vi "SL9200 Driver SM.vi"(0 "ComPort":refnum<visa-resource-name>="COM1", 2 "Mode":enum16{"Read", "Write"}(ring), 5 "Register":T1=49 items=["Heat_Flow", "Mass_Flow", "Corrected_Volume_Flow", "Volume_Flow", "Temperature", "Temperature2", "Delta_Temperature", "Pressure", "Diff_Pressure", "Density", "Spec_Enthalpy", "Date", "Time", "Level", "Peak_Demand", "Demand_Last_Hour", "Peak_Demand_Time", "Peak_Demand_Date", "Viscosity", "Reynolds_Number", "Heat_Total", "Grand_Heat_Total", "Mass_Total", "Grand_Mass", "Corrected_Volume_Total", "Grand_Corrected_Volume", "Volume_Total", "Grand_Volume", "Totalizer_Reset", "Alarm_Reset", "Barometric", "Fluid_Type", "Reference_Density", "Therm_Expansion_Coef", "Combustion_Heat", "Specific_Heat", "Flow_Z_Factor", "Ref_Z_Factor", "Isentropic_Exponent", "Viscosity_A", "Viscosity_B", "Reference_Temperature", "Calibration_Density", "Base_Density_H2O_4C", "Per_Mole_N2", "Per_Mole_CO2", "Tag_Number", "Software_Version", "Hardware_Version", "Order_Code", "Serial_Number", "Sensor_Serial_Num"], 7 "Write Data":string, 9 "InitSerial?":bool=TRUE, 11 "Error In":errorcluster, 12 "Close Com":bool) -> (4 "CMD OK":bool, 6 "Response":string, 15 "Error Out":errorcluster)   [LabVIEW 2016]
uses:
  Type Definitions/SL9200 Registers.ctl
  <vilib>/Instr/_visa.llb/VISA Configure Serial Port (Instr).vi
panel:
  out "Command String":string
  out "tStart":u32
  out "Time Array":i32[](array[numeric])
  out "State Array":string[](array[string])
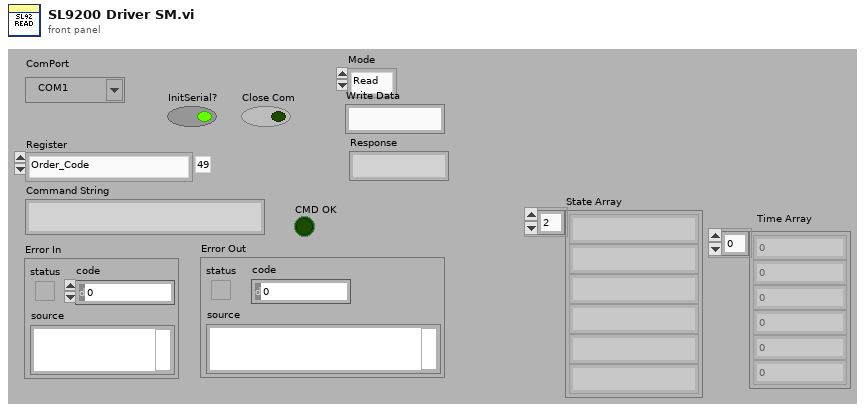
[diagram p1: front panel]
types:
  T1 = typedef "SL9200 Registers.ctl" = u8
  T2 = enum32{"invalid app kind", "Development System", "Run Time System", "Student Edition", "Embedded LabVIEW", "Evaluation", "Custom"}
  T3 = cluster{"Current VI Reference":refnum<vi>, "Close Panel on Exit?":bool}
  T4 = enum32{"Invalid", "Standard", "Closed", "Hidden", "Minimized", "Maximized"}
  T5 = cluster{"Core":cluster{"Current VI Reference":refnum<vi>, "Close Panel on Exit?":bool}, "ComPort":refnum<visa-resource-name>, "Response":string, "CMD OK":bool, "CMD":string, "Error Out Flag":bool}
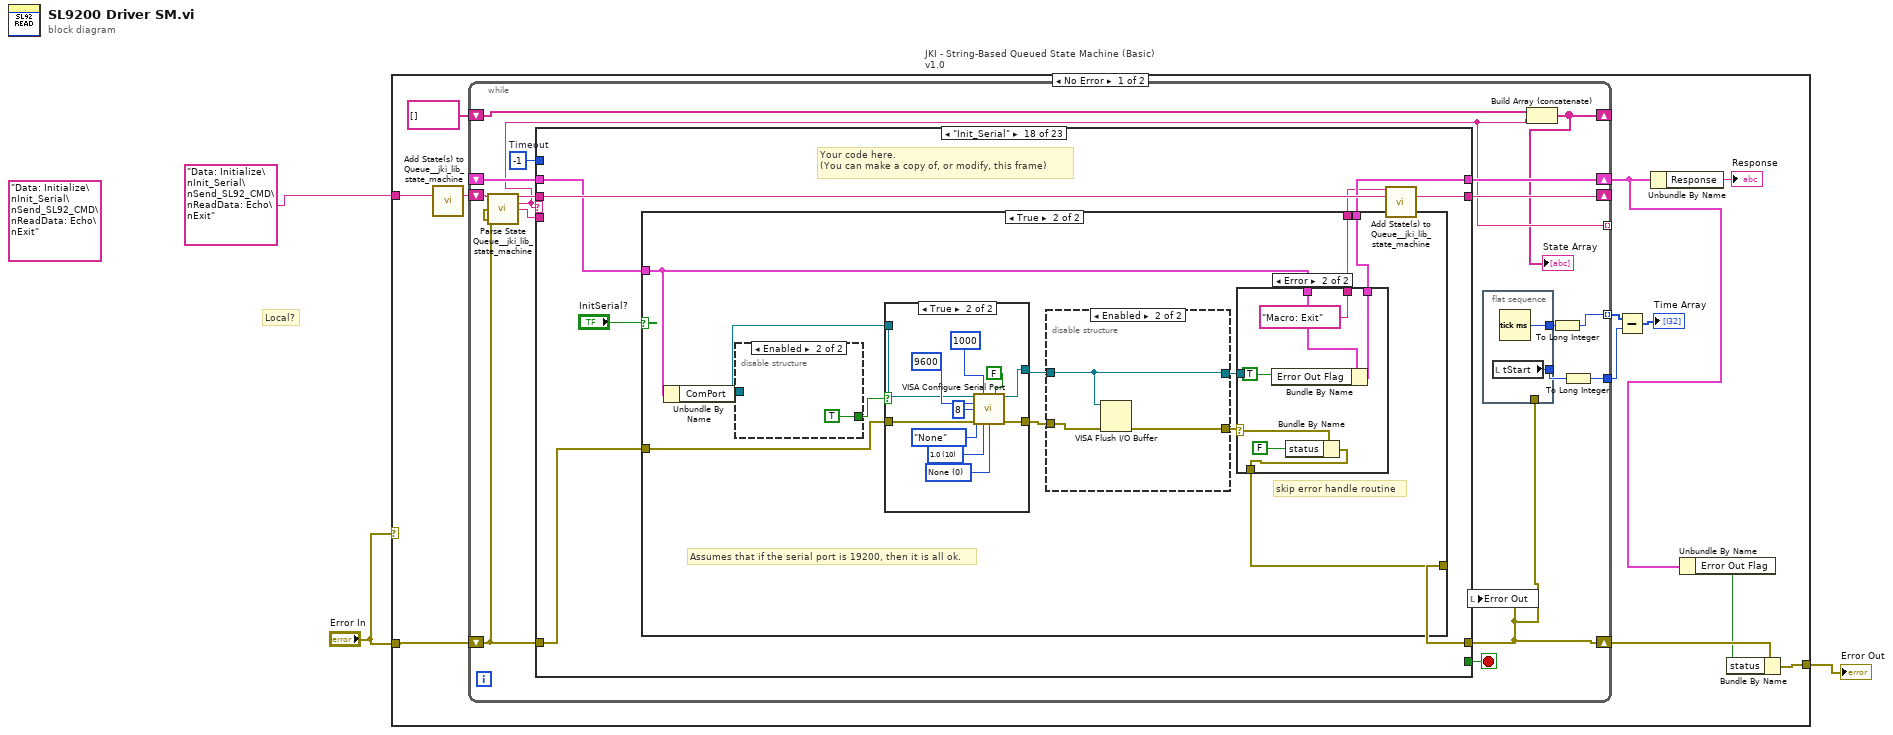
[diagram p0: block diagram]
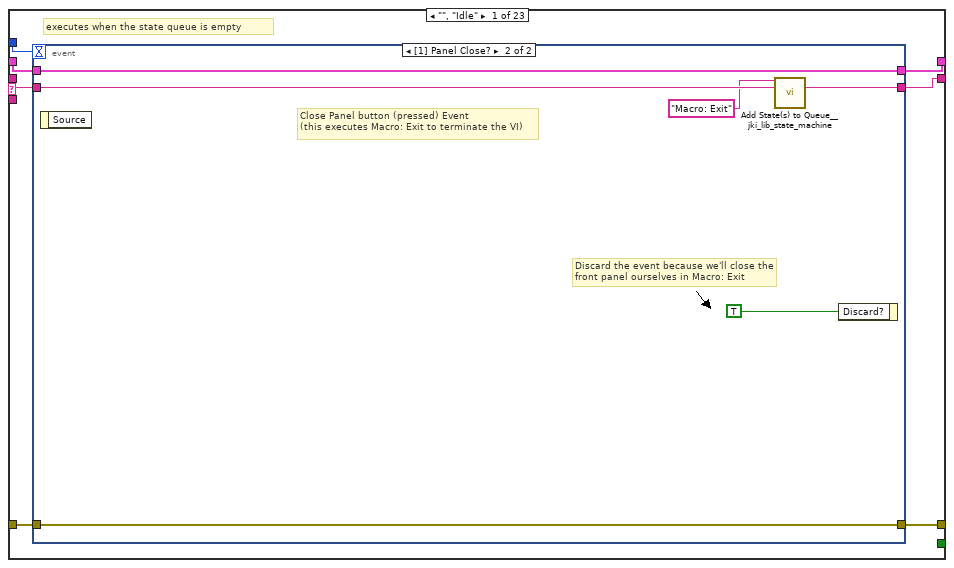
[diagram p2: hidden frame]
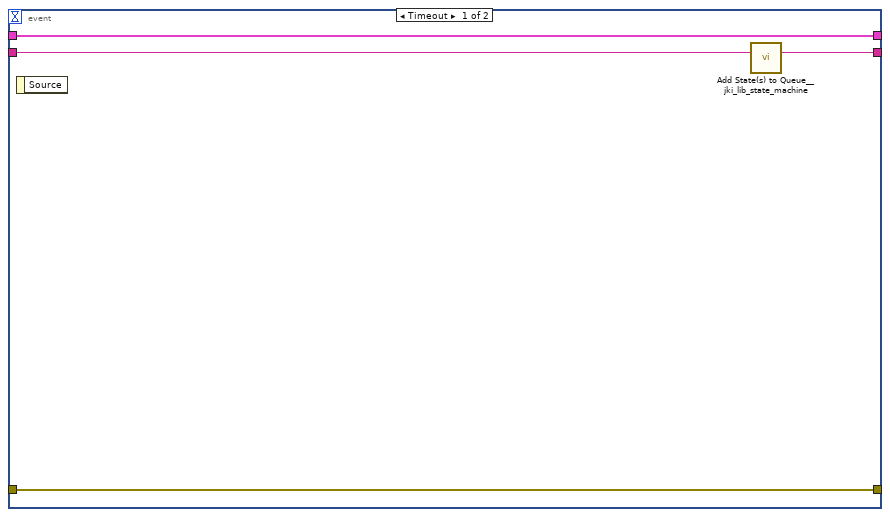
[diagram p3: hidden frame]
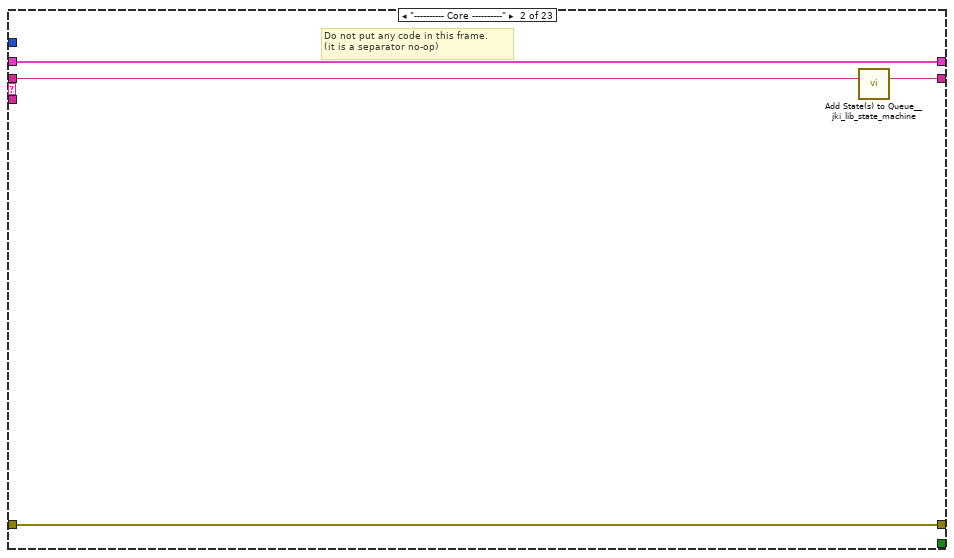
[diagram p4: hidden frame]
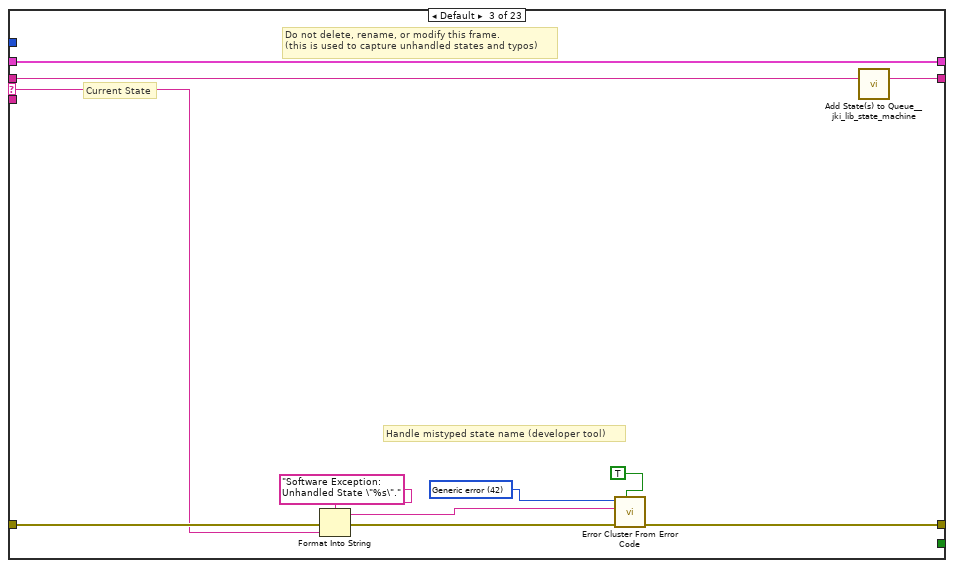
[diagram p5: hidden frame]
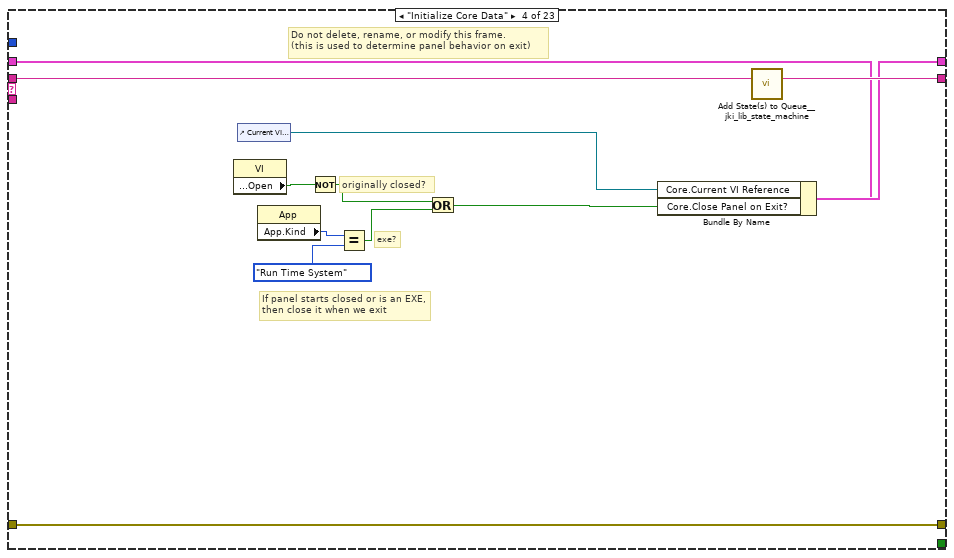
[diagram p6: hidden frame]
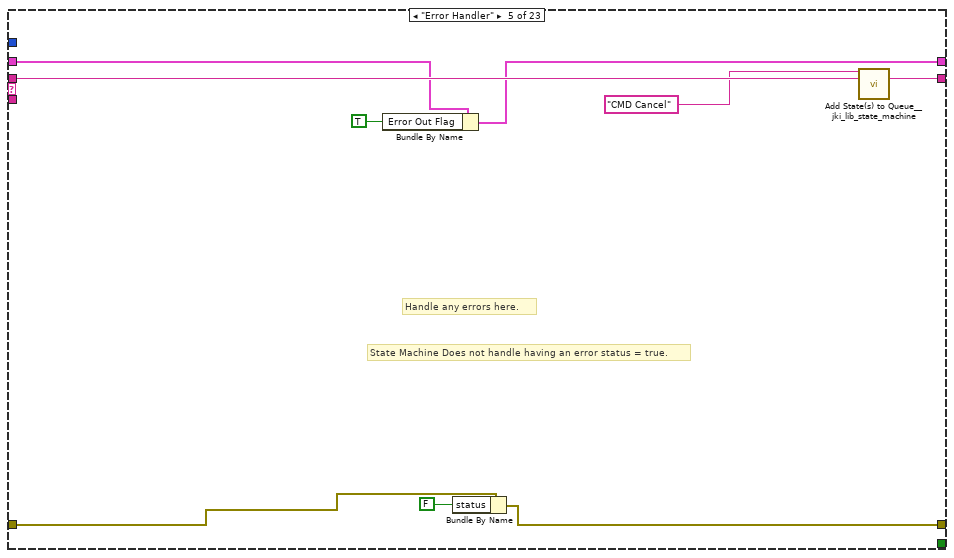
[diagram p7: hidden frame]
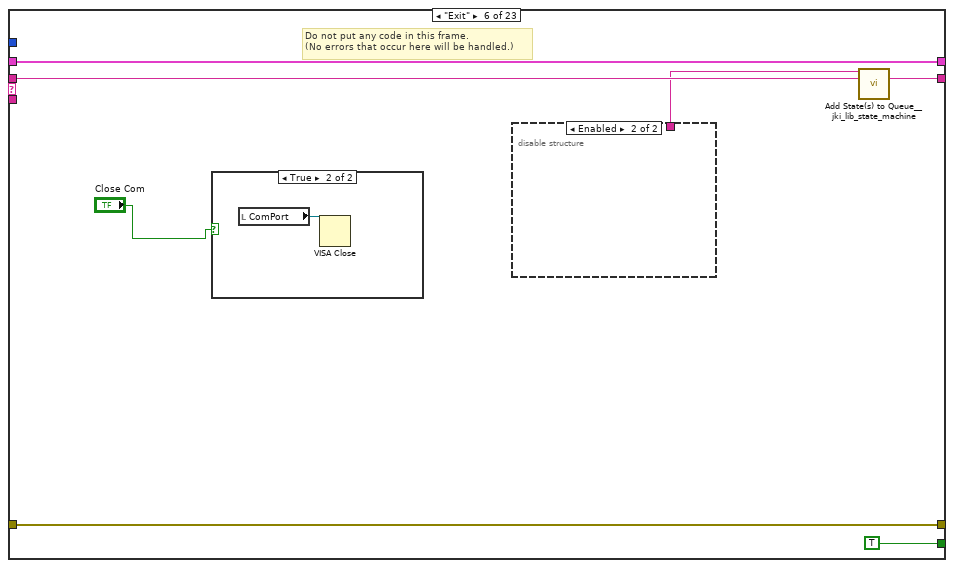
[diagram p8: hidden frame]
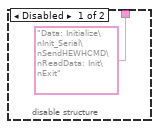
[diagram p10: hidden frame]
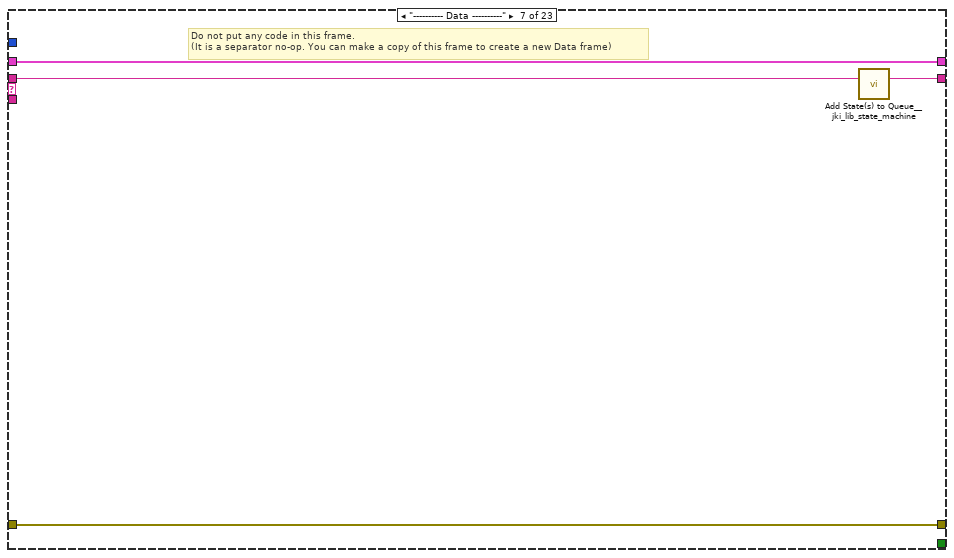
[diagram p11: hidden frame]
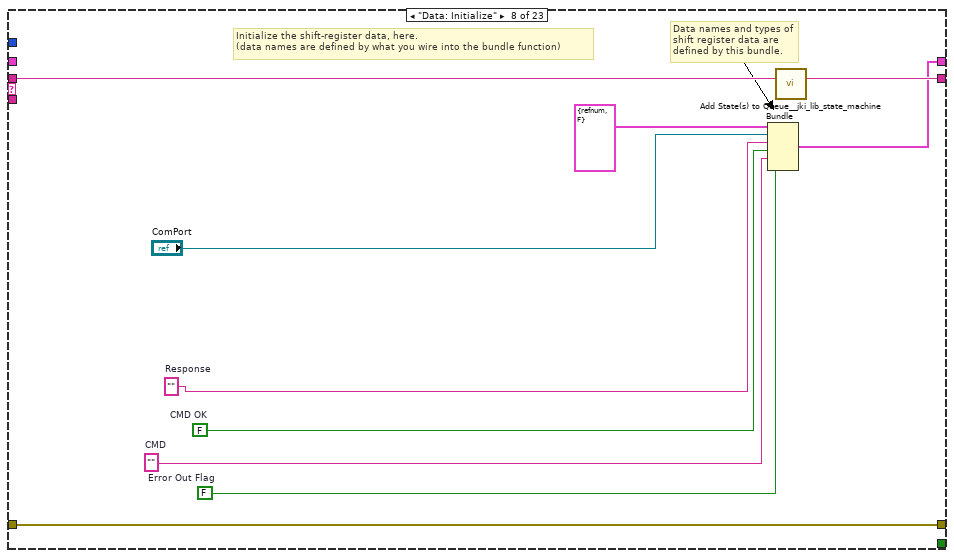
[diagram p12: hidden frame]
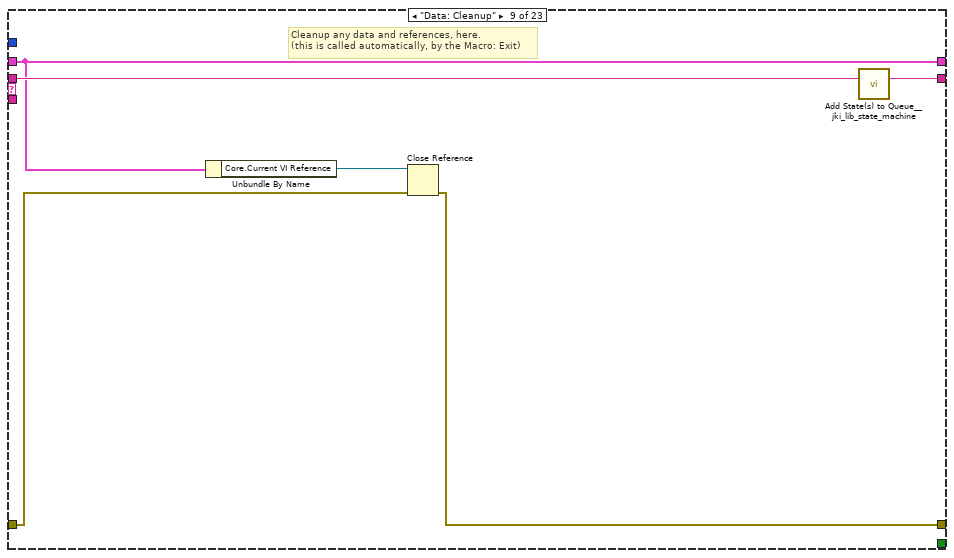
[diagram p13: hidden frame]
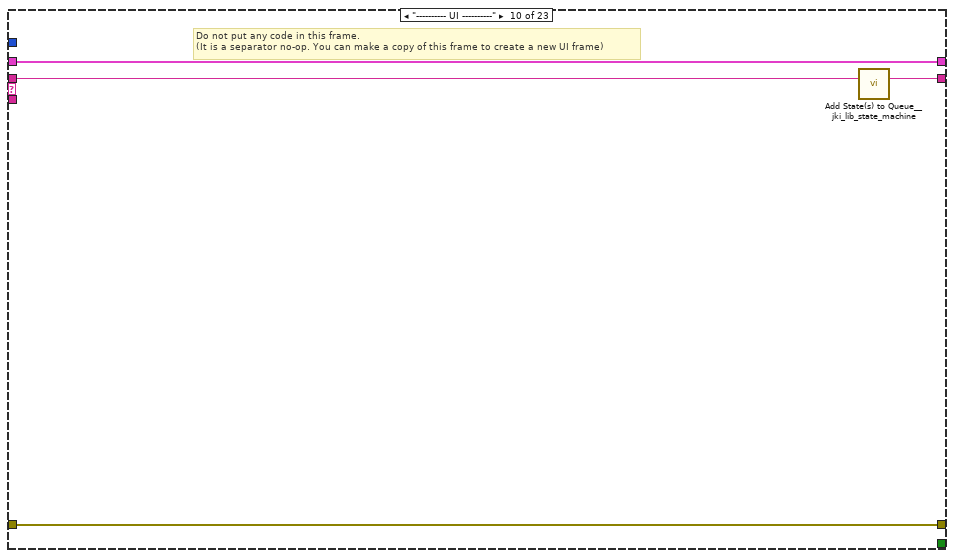
[diagram p14: hidden frame]
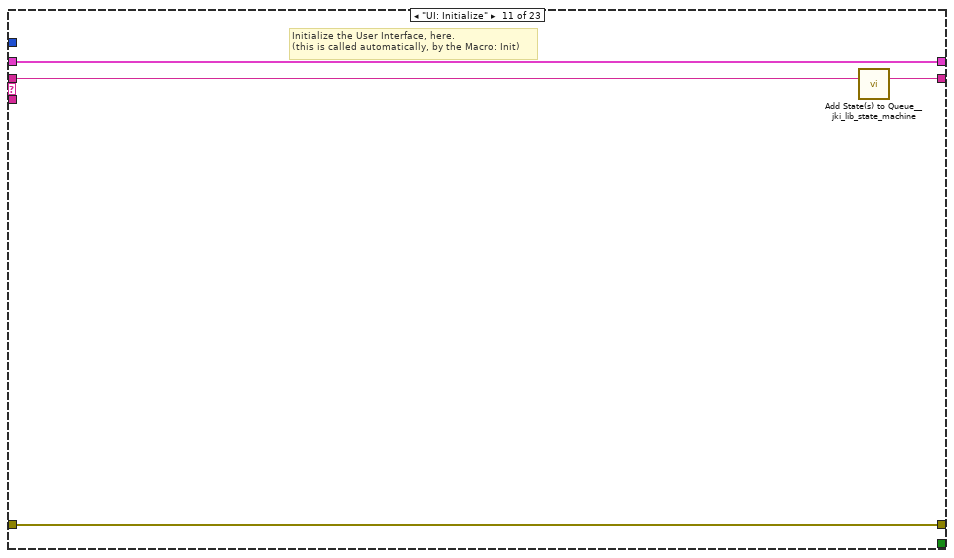
[diagram p15: hidden frame]
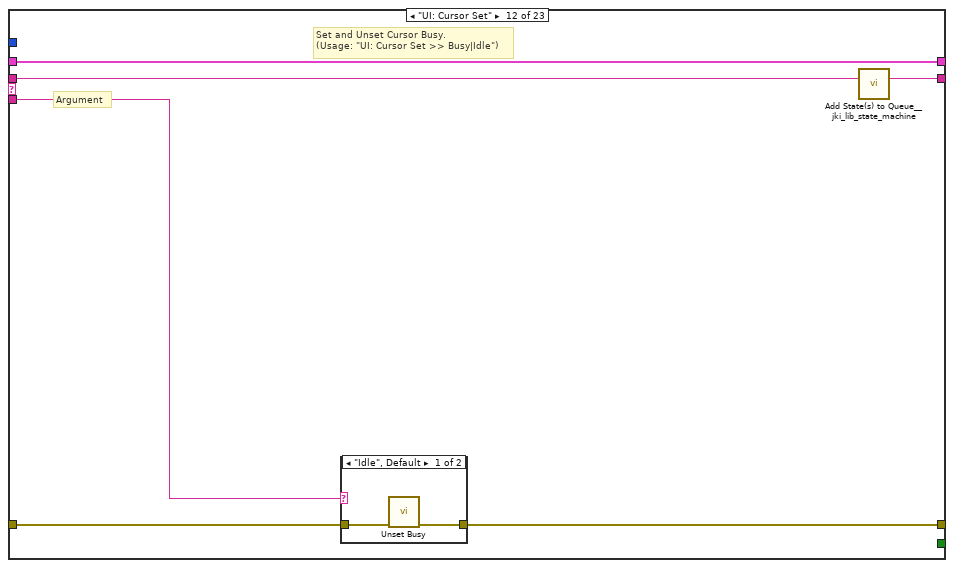
[diagram p16: hidden frame]
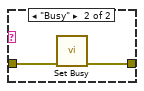
[diagram p17: hidden frame]
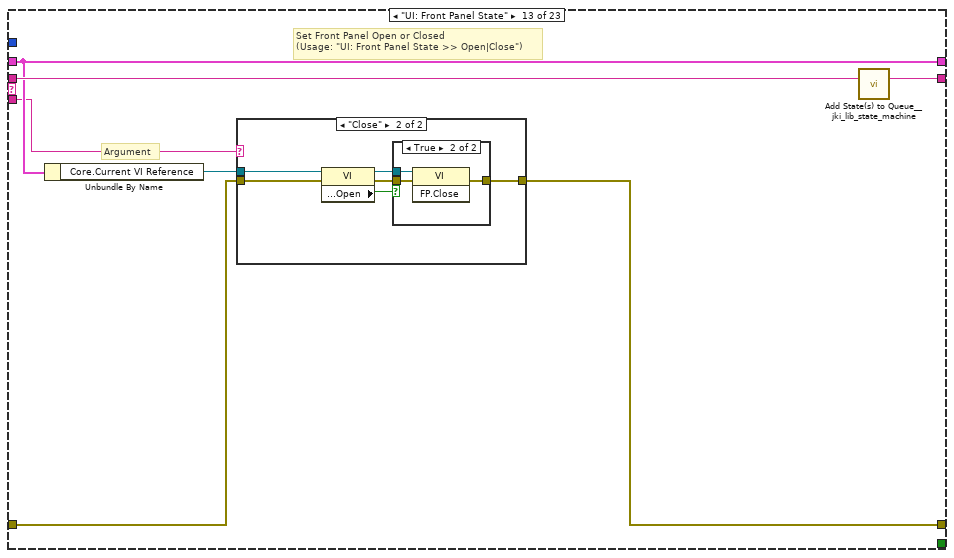
[diagram p18: hidden frame]
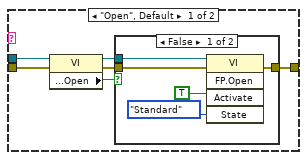
[diagram p19: hidden frame]
diagram:
  (unwired) "Data: Initialize\nInit_Serial\nSend_SL92_CMD\nReadData: Echo\nExit"
  # "Local?"
  n1 = case shown="No Error" "Error In" {
    tunnel: "Error In" -> [w14 w358]
    tunnel: [w8 w358] -> w3
    tunnel: "Data: Initialize\nInit_Serial\nSend_SL92_CMD\nReadData: Echo\nExit" -> [w4 _]
    frame No Error {
      n2 = call <vilib>:"Add State(s) to Queue__jki_lib_state_machine.vi"("State(s) in (\"\")"=w4) -> ("States Out"=w15:string)  [unwired: 14 in]
      n3 = while "JKI - String-Based Queued State Machine (Basic) v1.0" {
        shift-right: [w28] -> w7
        shift-left: _ -> [w27]
        shift-right: [w23] -> w13
        shift-left: w14 -> [w25]
        shift-right: [w24] -> _
        shift-left: w15 -> [w30]
        tunnel: [w17] -> _ mode=indexing
        tunnel: [w20] -> w11 mode=indexing
        tunnel: [w19] -> w10
        shift-right: [w16] -> _
        shift-left: string[] [] -> [w18]
        stop <- w29 stop-if-true
        w26 = -1  # Timeout
        n4 = call <vilib>:"Parse State Queue__jki_lib_state_machine.vi"("State Queue"=w30, "Error In (no error)"=w25) -> ("Remaining States"=w32:string, "Current State"=w17:string, "Arguments"=w31:string)  [unwired: 11 in]
        n5 = case shown="\"Init_Serial\"" w17 {
          selector: w17 -> [_ _ w56 _ _ _ _ _ _ _ _ _ _ _ _ _ _ _ _ _ _ _ _]
          tunnel: w32 -> [w41 w55 w60 w78 w87 w94 w100 w110 w116 w120 w124 w130 w141 w167 w172 w177 w188 w196 w295 w300 w312 w336 w357]
          tunnel: w31 -> [_ _ _ _ _ _ _ _ _ _ _ w125 w135 _ _ _ _ _ _ _ _ _ _]
          tunnel: w27 -> [w39 w52 w58 w69 w82 w92 w97 _ w113 w117 w122 w128 w137 w164 w169 w174 w185 w193 w290 w297 w308 w332 w350]
          tunnel: [w38 w53 w62 w75 w85 w91 w98 w107 w112 w118 w121 w126 w138 w165 w170 w175 w186 w194 w288 w298 w304 w329 w351] -> w23
          tunnel: w25 -> [w37 w53 w61 w75 w84 w91 w98 w107 w114 w118 w121 w127 w139 w165 w170 w175 w186 w191 w291 w298 w305 w330 w355]
          tunnel: [w40 w54 w59 w77 w86 w93 w99 w109 w115 w119 w123 w129 w140 w166 w171 w176 w187 w195 w294 w299 w311 w335 w356] -> w24
          tunnel: [_ _ _ _ _ TRUE _ _ _ _ _ _ _ _ _ _ _ _ _ _ _ _ _] -> w29
          tunnel: [w36 w52 w58 w76 w81 w92 w97 w108 w113 w117 w122 w128 w137 w164 w169 w174 w185 w192 w289 w297 w310 w334 w350] -> w28
          tunnel: w26 -> [w35 _ _ _ _ _ _ _ _ _ _ _ _ _ _ _ _ _ _ _ _ _ _]
          frame "", "Idle" {
            # "executes when the state queue is empty"
            n6 = event shown="[1] Panel Close?" {
              selector: _ -> [_ _]
              dyn-events: _ -> [_ _]
              timeout: w35 -> [_ _]
              tunnel: w41 -> [w45 w51]
              tunnel: [w44 w50] -> w40
              tunnel: w39 -> [w42 w48]
              tunnel: [w43 w49] -> w38
              tunnel: w37 -> [w43 w49]
              tunnel: [w42 w48] -> w36
              event Timeout {
                n7 = event-data() -> ()  [unwired: 1 in, 1 out]
                n8 = call <vilib>:"Add State(s) to Queue__jki_lib_state_machine.vi"("State(s) in (\"\")"=w45) -> ("States Out"=w44:string)  [unwired: 14 in]
              }
              event Panel Close? {
                # "Discard the event because we'll close the front panel ourselves in Macro: Exit"
                # "Close Panel button (pressed) Event\n(this executes Macro: Exit to terminate the VI)"
                n9 = event-data() -> ()  [unwired: 1 in, 1 out]
                n10 = call <vilib>:"Add State(s) to Queue__jki_lib_state_machine.vi"("State(s) in Front (\"\")"="Macro: Exit", "State(s) in (\"\")"=w51) -> ("States Out"=w50:string)  [unwired: 13 in]
                n11 = event-data("Discard?"=TRUE) -> ()  [unwired: 1 in, 1 out]
              }
            }
          }
          frame "---------- Core ----------" {
            # "Do not put any code in this frame.\n(it is a separator no-op)"
            n12 = call <vilib>:"Add State(s) to Queue__jki_lib_state_machine.vi"("State(s) in (\"\")"=w55) -> ("States Out"=w54:string)  [unwired: 14 in]
          }
          frame Default {
            w65 = 42 items=["No error", "Argument error", "Memory is full", "Out of zone", "End of file", "File already open", "Generic file I/O error", "File not found", "File permission error", "Disk is full", "Duplicate path", "Too many files open", "System feature not enabled", "Resource file not found", "Cannot add resource", "Resource not found", "Image not found", "Image memory error", "Pen does not exist", "Config type invalid", "Config token not found", "Config parse error", "Config memory error", "Bad external code format", "Bad external code offset", "External code not present", "Null window", "Destroy window error", "Null menu", "Print aborted", "Bad print record", "Print driver error", "Windows error during printing", "Memory error during printing", "Print dialog error", "Generic print error", "Invalid device refnum", "Device not found", "Device parameter error", "Device unit error", "Cannot open device", "Device call aborted", "Generic error", "Cancelled by user", "Object ID too low", "Object ID too high", "Object not in heap", "Unknown heap", "Unknown object (invalid DefProc)", "Unknown object (DefProc not in table)", "Message out of range", "Invalid (null) method", "Unknown message", "Manager call not supported", "Bad address", "Network operation in progress", "Network operation timed out", "Connection is busy", "Network attribute not supported", "Network error", "Address in use", "System out of memory", "Connection aborted", "Connection refused", "Not connected", "Already connected", "Connection closed", "Initialization error (interapplication manager)", "Bad occurrence", "Wait on unbound occurrence handler", "Occurrence queue overflow", "Datalog type conflict", "Unused", "Unrecognized type (interapplication manager)", "Memory corrupt", "Failed to make temporary DLL", "Old CIN version", "Drag socket not found", "Failed to load drop-object", "Failed to register OLE object", "Failed to release OLE object", "Format specifier type mismatch", "Unknown format specifier", "Too few format specifiers", "Too many format specifiers", "Scan failed", "Newer CIN version", "Error converting to variant", "Runtime menu error", "Password tampered", "Variant attribute not found", "Incompatible variant data type", "Event data is not available", "Event Store is not present", "Occurrence is not found", "Event Queue is not created", "Event info is not available", "Refnum passed is NULL", "Error retrieving Class GUID", "Error retrieving CoClass GUID", "Error retrieving TypeLib GUID.", "Bad built application magic bytes.", "Specific driver is different from the specific driver associated with the Logical Name.", "There is no session opened to the class driver.", "Max Error", "MAX - Error with config objects", "MAX - Error loading configuration", "MAX - Group not supported"]
            # "Current State"
            # "Do not delete, rename, or modify this frame.\n(this is used to capture unhandled states and typos)"
            # "Handle mistyped state name (developer tool)"
            n13 = Format Into String(format string="Software Exception: Unhandled State \"%s\"." ("message"), error in=w61, w56) -> (resulting string=w64:string, error out=w63:errorcluster)  [unwired: 1 in]
            n14 = call <vilib>:"Error Cluster From Error Code.vi"("show call chain? (False)"=TRUE, "error in (no error)"=w63, "error message (\"\")"=w64, "error code (0)"=w65) -> ("error out"=w62:errorcluster)  [unwired: 5 in]
            n15 = call <vilib>:"Add State(s) to Queue__jki_lib_state_machine.vi"("State(s) in (\"\")"=w60) -> ("States Out"=w59:string)  [unwired: 14 in]
          }
          frame "Initialize Core Data" {
            # "Do not delete, rename, or modify this frame.\n(this is used to determine panel behavior on exit)"
            # "originally closed?"
            # "exe?"
            # "If panel starts closed or is an EXE, then close it when we exit"
            n16 = property class="VI"() -> ("Front Panel.Open"=w74:bool)  [unwired: 2 in, 2 out]
            n17 = control-ref of="Current VI Reference"() -> (w67:refnum<vi>)
            n18 = property class="App"() -> ("App.Kind"=w73:T2)  [unwired: 2 in, 2 out]
            n19 = Not(x=w74) -> (.not. x?=w71:bool)
            n20 = Equal?(x=w73, y=T2."Run Time System" ("Application:Kind")) -> (x = y?=w70:bool)
            n21 = Or(x=w71, y=w70) -> (x .or. y?=w68:bool)
            n22 = Bundle By Name(cluster=w69, "Core.Current VI Reference"=w67, "Core.Close Panel on Exit?"=w68) -> (w76:T5)
            n23 = call <vilib>:"Add State(s) to Queue__jki_lib_state_machine.vi"("State(s) in (\"\")"=w78) -> ("States Out"=w77:string)  [unwired: 14 in]
          }
          frame "Error Handler" {
            # "State Machine Does not handle having an error status = true."
            # "Handle any errors here."
            n24 = Bundle By Name(cluster=w82, "Error Out Flag"=TRUE) -> (w81:T5)
            n25 = Bundle By Name(cluster=w84, "status"=FALSE) -> (w85:errorcluster)
            n26 = call <vilib>:"Add State(s) to Queue__jki_lib_state_machine.vi"("State(s) in Front (\"\")"="CMD Cancel", "State(s) in (\"\")"=w87) -> ("States Out"=w86:string)  [unwired: 13 in]
          }
          frame "Exit" {
            # "Do not put any code in this frame.\n(No errors that occur here will be handled.)"
            n27 = case shown="True" "Close Com" {
              frame False {
              }
              frame True {
                n28 = local read "ComPort"() -> (w95:refnum<visa-resource-name>)
                n29 = VISA Close(VISA resource name=w95) -> ()  [unwired: 1 in, 1 out]
              }
            }
            n30 = disable-structure shown="Enabled" {
              disable-tunnel: ["Data: Initialize\nInit_Serial\nSendHEWHCMD\nReadData: Init\nExit" _] -> w89
              frame Disabled {
              }
              frame Enabled {
              }
            }
            n31 = call <vilib>:"Add State(s) to Queue__jki_lib_state_machine.vi"("State(s) in Front (\"\")"=w89, "State(s) in (\"\")"=w94) -> ("States Out"=w93:string)  [unwired: 13 in]
          }
          frame "---------- Data ----------" {
            # "Do not put any code in this frame.\n(It is a separator no-op. You can make a copy of this frame to create a new Data frame)"
            n32 = call <vilib>:"Add State(s) to Queue__jki_lib_state_machine.vi"("State(s) in (\"\")"=w100) -> ("States Out"=w99:string)  [unwired: 14 in]
          }
          frame "Data: Initialize" {
            w101 = ""  # Response
            w102 = ""  # CMD
            w103 = FALSE  # Error Out Flag
            w105 = FALSE  # CMD OK
            # "Data names and types of shift register data are defined by this bundle."
            # "Initialize the shift-register data, here.\n(data names are defined by what you wire into the bundle function)"
            n33 = Bundle("Core"=T3 {"Current VI Reference"=refnum, "Close Panel on Exit?"=FALSE}, "ComPort"="ComPort", "Response"=w101, "CMD OK"=w105, "CMD"=w102, "Error Out Flag"=w103) -> (w108:T5)  [unwired: 1 in]
            n34 = call <vilib>:"Add State(s) to Queue__jki_lib_state_machine.vi"("State(s) in (\"\")"=w110) -> ("States Out"=w109:string)  [unwired: 14 in]
          }
          frame "Data: Cleanup" {
            # "Cleanup any data and references, here.\n(this is called automatically, by the Macro: Exit)"
            n35 = Unbundle By Name(w113) -> ("Core.Current VI Reference"=w111:refnum<vi>)
            n36 = Close Reference(reference=w111, error in (no error)=w114) -> (error out=w112:errorcluster)
            n37 = call <vilib>:"Add State(s) to Queue__jki_lib_state_machine.vi"("State(s) in (\"\")"=w116) -> ("States Out"=w115:string)  [unwired: 14 in]
          }
          frame "---------- UI ----------" {
            # "Do not put any code in this frame.\n(It is a separator no-op. You can make a copy of this frame to create a new UI frame)"
            n38 = call <vilib>:"Add State(s) to Queue__jki_lib_state_machine.vi"("State(s) in (\"\")"=w120) -> ("States Out"=w119:string)  [unwired: 14 in]
          }
          frame "UI: Initialize" {
            # "Initialize the User Interface, here.\n(this is called automatically, by the Macro: Init)"
            n39 = call <vilib>:"Add State(s) to Queue__jki_lib_state_machine.vi"("State(s) in (\"\")"=w124) -> ("States Out"=w123:string)  [unwired: 14 in]
          }
          frame "UI: Cursor Set" {
            # "Argument"
            # "Set and Unset Cursor Busy.\n(Usage: \"UI: Cursor Set >> Busy|Idle\")"
            n40 = case shown="\"Idle\", Default" w125 {
              tunnel: w127 -> [w132 w134]
              tunnel: [w131 w133] -> w126
              frame "Idle", Default {
                n41 = call <vilib>:"Unset Busy.vi"("error in (no error)"=w132) -> ("error out"=w131:errorcluster)  [unwired: 10 in]
              }
              frame "Busy" {
                n42 = call <vilib>:"Set Busy.vi"("error in (no error)"=w134) -> ("error out"=w133:errorcluster)  [unwired: 9 in, 1 out]
              }
            }
            n43 = call <vilib>:"Add State(s) to Queue__jki_lib_state_machine.vi"("State(s) in (\"\")"=w130) -> ("States Out"=w129:string)  [unwired: 14 in]
          }
          frame "UI: Front Panel State" {
            # "Argument"
            # "Set Front Panel Open or Closed\n(Usage: \"UI: Front Panel State >> Open|Close\")"
            n44 = Unbundle By Name(w137) -> ("Core.Current VI Reference"=w136:refnum<vi>)
            n45 = case shown="\"Close\"" w135 {
              tunnel: w139 -> [w145 w158]
              tunnel: [w147 w159] -> w138
              tunnel: w136 -> [w146 w156]
              frame "Open", Default {
                n46 = property class="VI"(reference=w146, error in=w145) -> (reference out=w143:refnum<vi>, error out=w144:errorcluster, "Front Panel.Open"=w142:bool)
                n47 = case shown="False" w142 {
                  tunnel: [w150 w153] -> w147
                  tunnel: w144 -> [w149 w153]
                  tunnel: w143 -> [w148 _]
                  frame False {
                    n48 = invoke class="VI" method="FP.Open"(reference=w148, error in=w149, "Activate"=TRUE, "State"=T4."Standard") -> (error out=w150:errorcluster)  [unwired: 1 in, 4 out]
                  }
                  frame True {
                  }
                }
              }
              frame "Close" {
                n49 = property class="VI"(reference=w156, error in=w158) -> (reference out=w155:refnum<vi>, error out=w157:errorcluster, "Front Panel.Open"=w154:bool)
                n50 = case shown="True" w154 {
                  tunnel: [w160 w163] -> w159
                  tunnel: w157 -> [w160 w162]
                  tunnel: w155 -> [_ w161]
                  frame False {
                  }
                  frame True {
                    n51 = invoke class="VI" method="FP.Close"(reference=w161, error in=w162) -> (error out=w163:errorcluster)  [unwired: 1 in, 2 out]
                  }
                }
              }
            }
            n52 = call <vilib>:"Add State(s) to Queue__jki_lib_state_machine.vi"("State(s) in (\"\")"=w141) -> ("States Out"=w140:string)  [unwired: 14 in]
          }
          frame "---------- Macro ----------" {
            # "Do not put any code in this frame.\n(It is a separator no-op. You can make a copy of this frame to create a new Macro frame)"
            n53 = call <vilib>:"Add State(s) to Queue__jki_lib_state_machine.vi"("State(s) in (\"\")"=w167) -> ("States Out"=w166:string)  [unwired: 14 in]
          }
          frame "Macro: Initialize" {
            w168 = "Data: Initialize\nInitialize Core Data\nUI: Initialize\nUI: Front Panel State >> Open\nInit_Serial"  # Data: Initialize Initialize Core Data UI: Initialize UI: Front Panel State >> Open Init_Serial
            # "Initialization Macro\n(This is called once, when the VI starts)"
            n54 = call <vilib>:"Add State(s) to Queue__jki_lib_state_machine.vi"("State(s) in Front (\"\")"=w168, "State(s) in (\"\")"=w172) -> ("States Out"=w171:string)  [unwired: 13 in]
          }
          frame "Macro: Exit" {
            # "Exit Macro\n(This is called once, when the VI exits)"
            n55 = disable-structure shown="Enabled" {
              disable-tunnel: w174 -> [w184 _]
              disable-tunnel: [w178 _] -> w173
              frame Enabled {
                n56 = Unbundle By Name(w184) -> ("Core.Close Panel on Exit?"=w183:bool)
                n57 = Select(t="UI: Front Panel State >> Close", s=w183, f="") -> (s? t:f=w180:string)
                n58 = call <vilib>:"Add State(s) to Queue__jki_lib_state_machine.vi"("State(s) in (\"\")"=w180, "State(s) at Back (\"\")"="Data: Cleanup\nExit") -> ("States Out"=w178:string)  [unwired: 13 in]
              }
              frame Disabled {
              }
            }
            n59 = call <vilib>:"Add State(s) to Queue__jki_lib_state_machine.vi"("State(s) in Front (\"\")"=w173, "State(s) in (\"\")"=w177) -> ("States Out"=w176:string)  [unwired: 13 in]
          }
          frame "---------- New Category ----------" {
            # "Template Separator\n(You can make a copy of, or modify, this frame)"
            n60 = call <vilib>:"Add State(s) to Queue__jki_lib_state_machine.vi"("State(s) in (\"\")"=w188) -> ("States Out"=w187:string)  [unwired: 14 in]
          }
          frame "Init_Serial" {
            # "Your code here.\n(You can make a copy of, or modify, this frame)"
            n61 = case shown="True" "InitSerial?" {
              tunnel: [w201 w223] -> w194
              tunnel: w193 -> [w200 w233]
              tunnel: [w199 w232] -> w192
              tunnel: w191 -> [w206 w226]
              tunnel: [w198 w224] -> w189
              frame False {
                # "skip error handle routine"
                n62 = Unbundle By Name(w200) -> ("ComPort"=w197:refnum<visa-resource-name>)
                n63 = property class="Instr"(reference=w197) -> (reference out=w203:refnum<visa-resource-name>, "Serial Settings:Number of Bytes at Serial Port"=w205:u32)  [unwired: 1 in, 1 out]
                n64 = Greater Than 0?(x=w205) -> (x > 0?=w204:bool)
                n65 = case shown="True" w204 {
                  tunnel: w206 -> [w219 w222]
                  tunnel: [w219 w221] -> w202
                  tunnel: w203 -> [_ w220]
                  frame False {
                  }
                  frame True {
                    n66 = VISA Clear(VISA resource name=w220, error in (no error)=w222) -> (error out=w221:errorcluster)  [unwired: 1 out]
                  }
                }
                n67 = case shown="No Error" w202 {
                  selector: w202 -> [w207 w214]
                  tunnel: w200 -> [w211 w218]
                  tunnel: [w210 w217] -> w199
                  tunnel: w197 -> [w209 _]
                  tunnel: ["" ("State(s) in Front (\"\")") "Macro: Exit" ("State(s) in Front (\"\")")] -> w198
                  tunnel: [w207 w213] -> w201
                  frame No Error {
                    n68 = Bundle By Name(cluster=w211, "ComPort"=w209) -> (w210:T5)
                  }
                  frame Error {
                    n69 = Bundle By Name(cluster=w218, "Error Out Flag"=TRUE) -> (w217:T5)
                    n70 = Bundle By Name(cluster=w214, "status"=FALSE) -> (w213:errorcluster)
                  }
                }
              }
              frame True {
                # "skip error handle routine"
                # "Assumes that if the serial port is 19200, then it is all ok."
                n71 = Unbundle By Name(w233) -> ("ComPort"=w231:refnum<visa-resource-name>)
                n72 = disable-structure shown="Enabled" {
                  disable-tunnel: w231 -> [w269 _]
                  disable-tunnel: [w266 TRUE] -> w230
                  frame Disabled {
                    n73 = property class="Instr"(reference=w269) -> ("Baud"=w268:u32)  [unwired: 1 in, 2 out]
                    n74 = Not Equal?(x=w268, y=u32 19200) -> (x != y?=w266:bool)
                  }
                  frame Enabled {
                  }
                }
                n75 = case shown="True" w230 {
                  tunnel: [w271 w274] -> w229
                  tunnel: [w272 w273] -> w227
                  tunnel: w226 -> [w271 w276]
                  tunnel: w231 -> [w272 w275]
                  frame False {
                  }
                  frame True {
                    w282 = u16 0 items=["None", "XON/XOFF", "RTS/CTS", "XON/XOFF & RTS/CTS", "DTR/DSR", "XON/XOFF & DTR/DSR"] ("flow control (0:none)")
                    w281 = u16 10 items=["1.0"=10, "1.5"=15, "2.0"=20] ("stop bits (10: 1 bit)")
                    n76 = call-poly "VISA Configure Serial Port"("VISA resource name"=w275, "timeout (10sec)"=u32 1000, "Enable Termination\nChar (T)"=FALSE ("Enable Termination\nChar (T)"), "baud rate (9600)"=u32 9600, "data bits (8)"=u16 8, "parity (0:none)"=enum16{"None", "Odd", "Even", "Mark", "Space"}."None", "error in (no error)"=w276, "stop bits (10: 1 bit)"=w281, "flow control (0:none)"=w282) -> ("VISA resource name out"=w273:refnum<visa-resource-name>, "error out"=w274:errorcluster)  [unwired: 5 in]
                  }
                }
                n77 = disable-structure shown="Enabled" {
                  disable-tunnel: w229 -> [w251 w265]
                  disable-tunnel: [w250 w264] -> w225
                  disable-tunnel: [w249 w263] -> w228
                  disable-tunnel: w227 -> [w248 w263]
                  frame Disabled {
                    n78 = disable-structure shown="Enabled" {
                      disable-tunnel: w248 -> [w254 w256]
                      disable-tunnel: [w253 w256] -> w247
                      disable-tunnel: [w252 u32 1 ("Bytes at Port")] -> w246
                      frame Disabled {
                        n79 = property class="Instr"(reference=w254) -> (reference out=w253:refnum<visa-resource-name>, "Serial Settings:Number of Bytes at Serial Port"=w252:u32)  [unwired: 1 in, 1 out]
                      }
                      frame Enabled {
                      }
                    }
                    n80 = case shown="1, Default" w246 {
                      tunnel: w251 -> [w258 w262]
                      tunnel: [w258 w261] -> w250
                      tunnel: [w257 w260] -> w249
                      tunnel: w247 -> [w257 w259]
                      frame 0 {
                      }
                      frame 1, Default {
                        n81 = VISA Clear(VISA resource name=w259, error in (no error)=w262) -> (VISA resource name out=w260:refnum<visa-resource-name>, error out=w261:errorcluster)
                      }
                    }
                  }
                  frame Enabled {
                    n82 = VISA Flush I/O Buffer(VISA resource name=w263, error in (no error)=w265) -> (error out=w264:errorcluster)  [unwired: 1 in, 1 out]
                  }
                }
                n83 = case shown="Error" w225 {
                  selector: w225 -> [w234 w241]
                  tunnel: w233 -> [w238 w245]
                  tunnel: [w237 w244] -> w232
                  tunnel: w228 -> [w236 _]
                  tunnel: ["" ("State(s) in Front (\"\")") "Macro: Exit" ("State(s) in Front (\"\")")] -> w224
                  tunnel: [w234 w239] -> w223
                  frame No Error {
                    n84 = Bundle By Name(cluster=w238, "ComPort"=w236) -> (w237:T5)
                  }
                  frame Error {
                    n85 = Bundle By Name(cluster=w245, "Error Out Flag"=TRUE) -> (w244:T5)
                    n86 = Bundle By Name(cluster=w241, "status"=FALSE) -> (w239:errorcluster)
                  }
                }
              }
            }
            n87 = call <vilib>:"Add State(s) to Queue__jki_lib_state_machine.vi"("State(s) in Front (\"\")"=w189, "State(s) in (\"\")"=w196) -> ("States Out"=w195:string)  [unwired: 13 in]
          }
          frame "Send_SL92_CMD" {
            n88 = call "SL9200 CMD.vi"("Mode"="Mode", "Command"="Register", "Write Data"="Write Data") -> ("Command String"=w287:string)  [unwired: 12 in]
            "Command String" <- w287
            n89 = Unbundle By Name(w290) -> ("ComPort"=w293:refnum<visa-resource-name>)
            n90 = VISA Write(VISA resource name=w293, write buffer=w287, error in (no error)=w291) -> (error out=w288:errorcluster)  [unwired: 2 out]
            n91 = flat-sequence {
              tunnel: [w296] -> w292
              tunnel: w291 -> [_]
              frame #0 {
                n92 = Tick Count (ms)() -> (millisecond timer value=w296:u32)
              }
            }
            n93 = Bundle By Name(cluster=w290, "CMD"=w287) -> (w289:T5)
            n94 = call <vilib>:"Add State(s) to Queue__jki_lib_state_machine.vi"("State(s) in (\"\")"=w295) -> ("States Out"=w294:string)  [unwired: 14 in]
            "tStart" <- w292
          }
          frame " ------- ReadData ------------ " {
            # "Template Separator\n(You can make a copy of, or modify, this frame)"
            n95 = call <vilib>:"Add State(s) to Queue__jki_lib_state_machine.vi"("State(s) in (\"\")"=w300) -> ("States Out"=w299:string)  [unwired: 14 in]
          }
          frame "ReadData: Echo" {
            # "Your code here.\n(You can make a copy of, or modify, this frame)"
            n96 = Unbundle By Name(w308) -> ("CMD"=w302:string, "ComPort"=w307:refnum<visa-resource-name>)
            n97 = while {
              tunnel: w307 -> [w325]
              shift-right: [w323] -> w303
              shift-left: "" -> [w322]
              shift-right: [w315] -> w304
              shift-left: w305 -> [w321]
              stop <- w317 stop-if-true
              n98 = VISA Read(VISA resource name=w325, byte count=u32 1, error in (no error)=w321) -> (read buffer=w320:string, error out=w315:errorcluster)  [unwired: 2 out]
              n99 = Equal?(x=w320, y="\r") -> (x = y?=w316:bool)
              n100 = Concatenate Strings(w322, w320) -> (w323:string)
              n101 = Unbundle By Name(w315) -> ("status"=w318:bool)
              n102 = Or(x=w316, y=w318) -> (x .or. y?=w317:bool)
            }
            n103 = Equal?(x=w302, y=w303) -> (x = y?=w301:bool)
            "CMD OK" <- w301
            n104 = Bundle By Name(cluster=w308, "CMD OK"=w301) -> (w310:T5)
            n105 = case shown="False" w301 {
              tunnel: ["CMD Cancel" ("State(s) in Front (\"\")") "ReadData: Response" ("State(s) in Front (\"\")")] -> w309
              frame False {
              }
              frame True {
              }
            }
            n106 = call <vilib>:"Add State(s) to Queue__jki_lib_state_machine.vi"("State(s) in Front (\"\")"=w309, "State(s) in (\"\")"=w312) -> ("States Out"=w311:string)  [unwired: 13 in]
          }
          frame "ReadData: Response" {
            n107 = Unbundle By Name(w332) -> ("ComPort"=w326:refnum<visa-resource-name>)  [unwired: 1 out]
            n108 = while {
              tunnel: w326 -> [w349]
              shift-right: [w347] -> w328
              shift-left: "" -> [w346]
              shift-right: [w340] -> w329
              shift-left: w330 -> [w345]
              tunnel: [w339] -> w327
              stop <- w341 stop-if-true
              n109 = VISA Read(VISA resource name=w349, byte count=u32 1, error in (no error)=w345) -> (read buffer=w344:string, error out=w340:errorcluster)  [unwired: 2 out]
              n110 = Equal?(x=w344, y="\n") -> (x = y?=w339:bool)
              n111 = Concatenate Strings(w346, w344) -> (w347:string)
              n112 = Unbundle By Name(w340) -> ("status"=w342:bool)
              n113 = Or(x=w339, y=w342) -> (x .or. y?=w341:bool)
            }
            n114 = Bundle By Name(cluster=w332, "Response"=w328) -> (w334:T5)
            n115 = case shown="False" w327 {
              tunnel: ["CMD Cancel\nExit" ("State(s) in Front (\"\")") "Exit" ("State(s) in Front (\"\")")] -> w333
              frame False {
              }
              frame True {
              }
            }
            n116 = call <vilib>:"Add State(s) to Queue__jki_lib_state_machine.vi"("State(s) in Front (\"\")"=w333, "State(s) in (\"\")"=w336) -> ("States Out"=w335:string)  [unwired: 13 in]
          }
          frame "CMD Cancel" {
            n117 = Unbundle By Name(w350) -> ("ComPort"=w354:refnum<visa-resource-name>)
            n118 = Byte Array To String(unsigned byte array=u8[] [27, 13]) -> (string=w352:string)
            n119 = VISA Write(VISA resource name=w354, write buffer=w352, error in (no error)=w355) -> (error out=w351:errorcluster)  [unwired: 2 out]
            n120 = call <vilib>:"Add State(s) to Queue__jki_lib_state_machine.vi"("State(s) in (\"\")"=w357) -> ("States Out"=w356:string)  [unwired: 14 in]
          }
        }
        n121 = local write "Error Out"(w23) -> ()
        n122 = flat-sequence {
          tunnel: [w34] -> w22
          tunnel: w23 -> [_]
          tunnel: [w33] -> w21
          frame #0 {
            n123 = local read "tStart"() -> (w33:u32)
            n124 = Tick Count (ms)() -> (millisecond timer value=w34:u32)
          }
        }
        n125 = Build Array (concatenate)(w18, w17) -> (w16:string[])
        "State Array" <- w16
        n126 = To Long Integer(number=w22) -> (32bit integer=w20:i32)
        n127 = To Long Integer(number=w21) -> (32bit integer=w19:i32)
      }
      n128 = Subtract(x=w11, y=w10) -> (x-y=→"Time Array":i32[])
      n129 = Unbundle By Name(w7) -> ("Response"=→"Response":string)
      n130 = Unbundle By Name(w7) -> ("Error Out Flag"=w6:bool)
      n131 = Bundle By Name(cluster=w13, "status"=w6) -> (w8:errorcluster)
    }
    frame Error {
    }
  }
  "Error Out" <- w3
